vi "Single Axis Tuner.vi"() -> ()   [LabVIEW 2010]
doc: "Motor testing and tuning application for NI-73xx motion controllers. Change control loop gains, software limits, home voltage position, and other axis specific parameters on the fly for up to eight axes.\n\nDependencies:\n\nfindHome.vi\nRead Joint Angle.vi\nRead Pot.vi"
uses:
  Shared/typedefs/Trajectory Parameters.ctl
  <vilib>/Motion/FlexMotion/CustomControls/CustomControls.llb/Resource Out (Enum).flx
  <vilib>/Utility/error.llb/DialogType.ctl
  <vilib>/Motion/FlexMotion/CustomControls/CustomControls.llb/ControlGainParameter.flx
  <vilib>/Motion/FlexMotion/FunctionsVIs/StartStopMotion.llb/Stop Motion (8 axes).flx
panel:
  in  "Home Accel (RPS/s)":dbl=4.0 format="%.2f"
  in  "Home Velocity (RPM)":i32=65
  in  "Target Positions (Encoder Counts)":i32[](array[numeric])
  in  "Plot Offset":i32 step=500
  in  "Stop Type":u16(ring) items=["Decelerate", "Halt", "Kill"]
  in  "Board ID":T1=1 min=1 max=32 step=1
  in  "Reset Position":bool
  in  "Repeat Move":bool
  out "Encoder Position":i32
  out "Status Indicators":T2
  out "Desired and Actual Position v Time":T3(graph)
  out "Velocity v Time":cluster{dbl, "Position":i32}[](graph)
  out "Last Velocity":i32
  out "Last Following Error":i16=32767
  out "Following Error v Time":cluster{dbl, "Following Error":i32}[](graph)
  out "RMS Following Error":dbl
  out "Pot Value":dbl format="%#_4g"
  out "Pot Slider":dbl(slide) scale=0.0..5.0
  in  "Home Position":dbl=2.626 caption="Volts"
  in  "Axis":T4=1 items=["Axis Control"=0, "Axis 1"=1, "Axis 2"=2, "Axis 3"=3, "Axis 4"=4, "Axis 5"=5, "Axis 6"=6, "Axis 7"=7, "Axis 8"=8, "Vector Space Control"=16, "Vector Space 1"=17, "Vector Space 2"=18, "Vector Space 3"=19, "Vector Space 4"=20, "Encoder Control"=32, "Encoder 1"=33, "Encoder 2"=34, "Encoder 3"=35, "Encoder 4"=36, "Encoder 5"=37, "Encoder 6"=38, "Encoder 7"=39, "Encoder 8"=40, "DAC Channel 1"=49, "DAC Channel 2"=50, "DAC Channel 3"=51, "DAC Channel 4"=52, "DAC Channel 5"=53, "DAC Channel 6"=54, "DAC Channel 7"=55, "DAC Channel 8"=56, "Stepper Output 1"=65, "Stepper Output 2"=66, "Stepper Output 3"=67, "Stepper Output 4"=68, "Stepper Output 5"=69, "Stepper Output 6"=70, "Stepper Output 7"=71, "Stepper Output 8"=72, "ADC Channel 1"=81, "ADC Channel 2"=82, "ADC Channel 3"=83, "ADC Channel 4"=84, "ADC Channel 5"=85, "ADC Channel 6"=86, "ADC Channel 7"=87, "ADC Channel 8"=88]
  in  "Reverse SW Limit":i32=-27000 caption="Counts"
  in  "Forward SW Limit":i32=27000 caption="Counts"
  in  "Go Home":bool
  in  "Kill":bool
  in  "end program":bool
  in  "Control Gains":cluster{"Kp":u16, "Ki":u16, "Kd":u16}={"Kp"=25, "Ki"=3, "Kd"=7000}
  in  "Start":bool
  in  "Trajectory Parameters":T5={"Operation Mode (Absolute)"=0, "Blend"=FALSE, "Velocity"=6.0, "Acceleration"=4.0, "Deceleration"=4.0, "Blend Factor"=0, "Permitted Following Error"=1000.0, "S Curve Time"=0} {"Operation Mode (Absolute)" items=["Absolute Position", "Relative Position"]; "Velocity" min=0.0 max=500.0 step=1.0}
  # "NOTE: Set Board ID before beginning program execution"
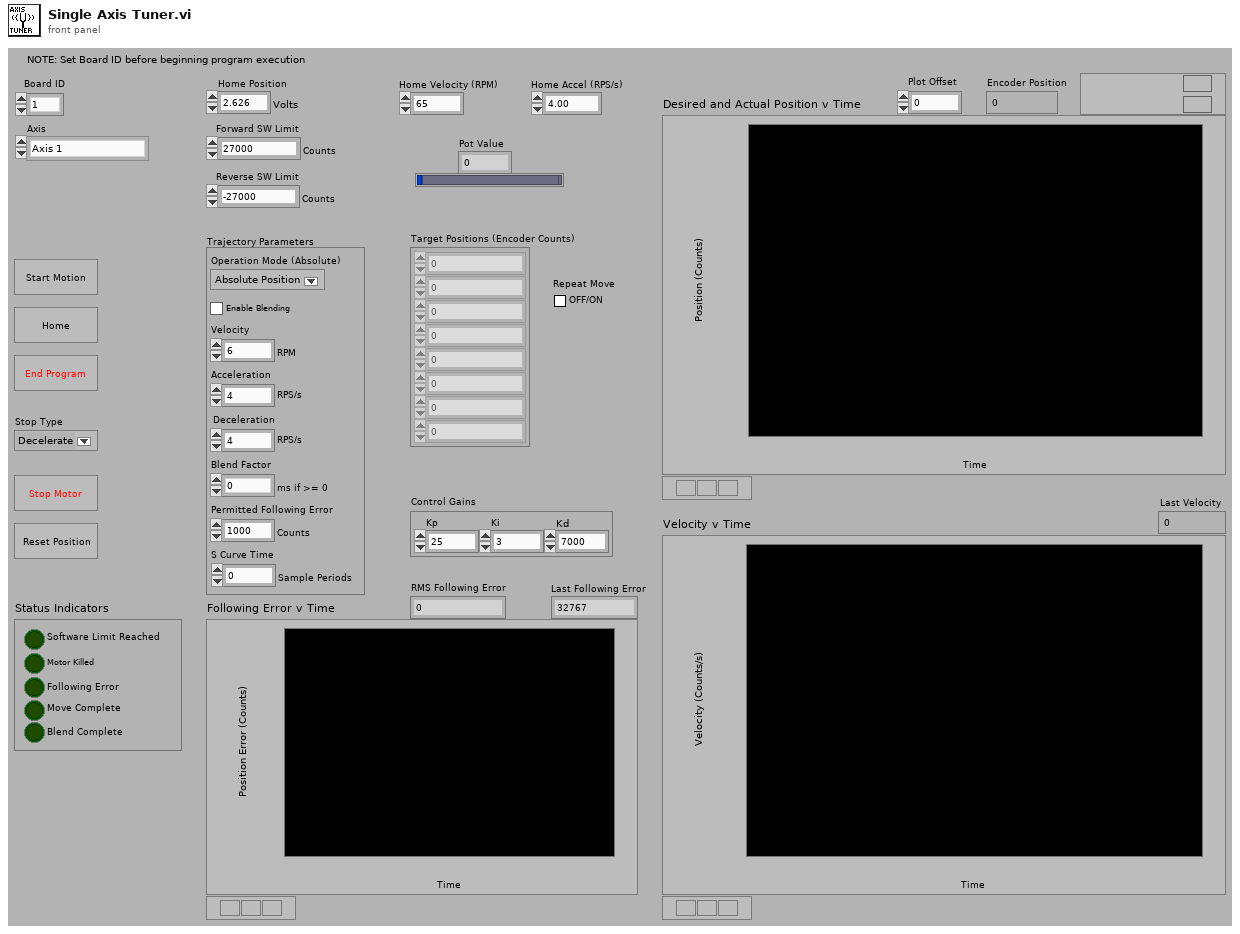
[diagram p1: front panel]
types:
  T1 = typedef "Board Id" = u8
  T2 = cluster{"Software Limit Reached":bool, "Motor Killed":bool, "Following Error":bool, "Move Complete":bool, "Blend Complete":bool}
  T3 = cluster{cluster{dbl, "Encoder Position":i32}[]}[]
  T4 = typedef "Resource Out (Enum).flx" = u16
  T5 = typedef "Trajectory Parameters.ctl" = cluster{"Operation Mode (Absolute)":u16, "Blend":bool, "Velocity":dbl, "Acceleration":dbl, "Deceleration":dbl, "Blend Factor":i16, "Permitted Following Error":dbl, "S Curve Time":u16}
  T6 = typedef "DialogType.ctl" = u16
  T7 = typedef "Bd Id Out" = u8
  T8 = cluster{"Ready to Receive":bool, "Return Data Pending":bool, "Reserved":bool, "CIP":bool, "Packet Error":bool, "Power Up Reset":bool, "Error Message":bool, "Hardware Fail":bool}
  T9 = typedef "ControlGainParameter.flx" = enum16{"Kp", "Ki", "IL", "Kd", "Td", "Kv", "Aff", "Vff"}
  T10 = enum8{"Enabled", "Disabled", "Disabled and Grayed Out"}
  T11 = typedef "Axis To Control.flx" = u16
  T12 = cluster{"Run/Stop":bool, "Profile Complete":bool, "Motor Off ":bool, "Following Error":bool, "Limit Switch":bool, "Home Switch":bool, "SW Limit Switch":bool, "Watchdog":bool, "Velocity Threshold":bool, "Position Brkpt":bool, "Home Found":bool, "Index Found":bool, "High Speed Capture":bool, "Reverse Direction":bool, "Blend Complete":bool, "Move Complete":bool}
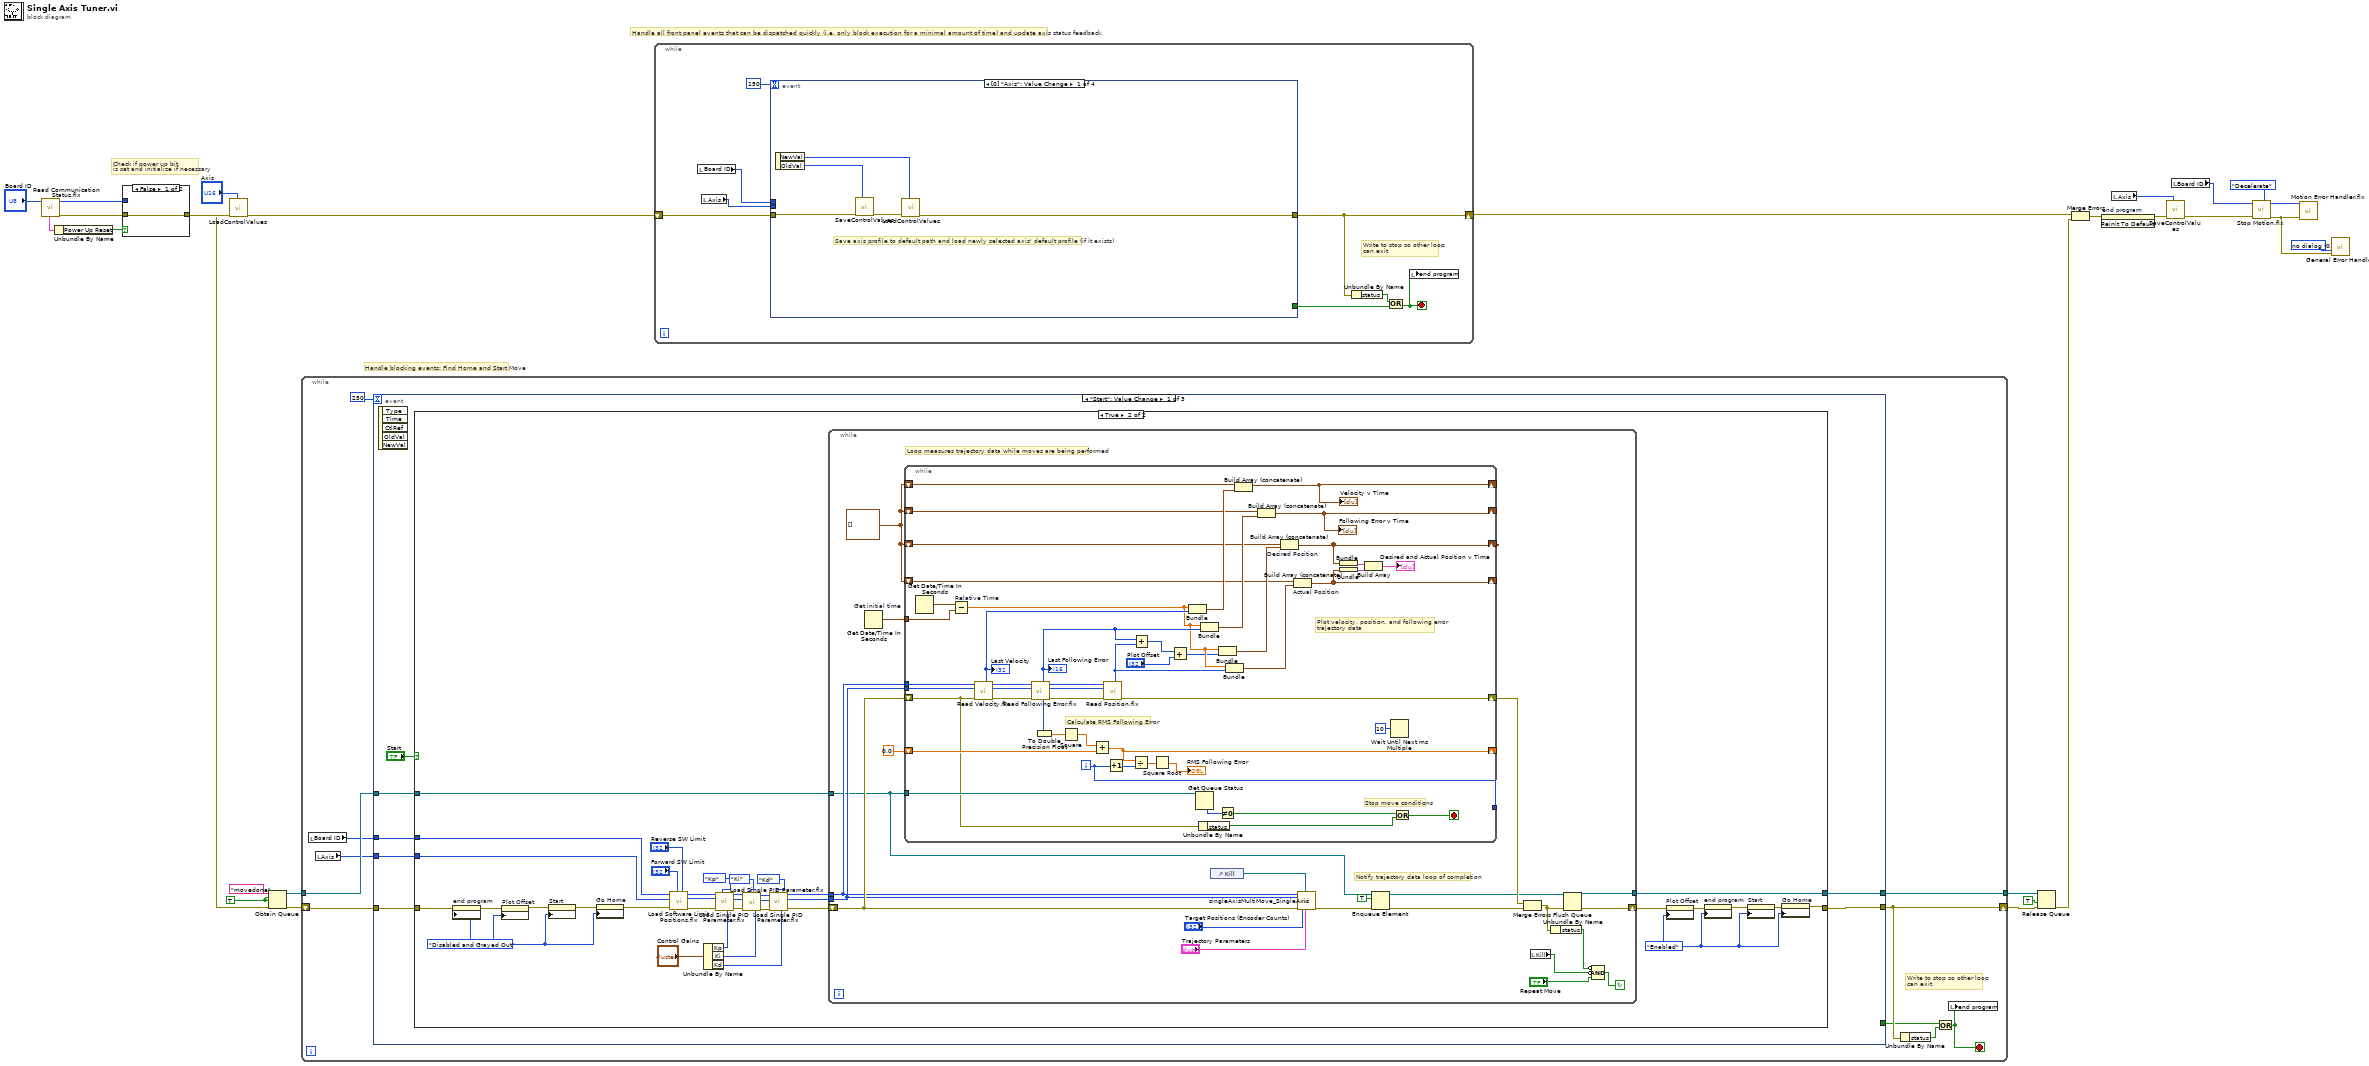
[diagram p0: block diagram]
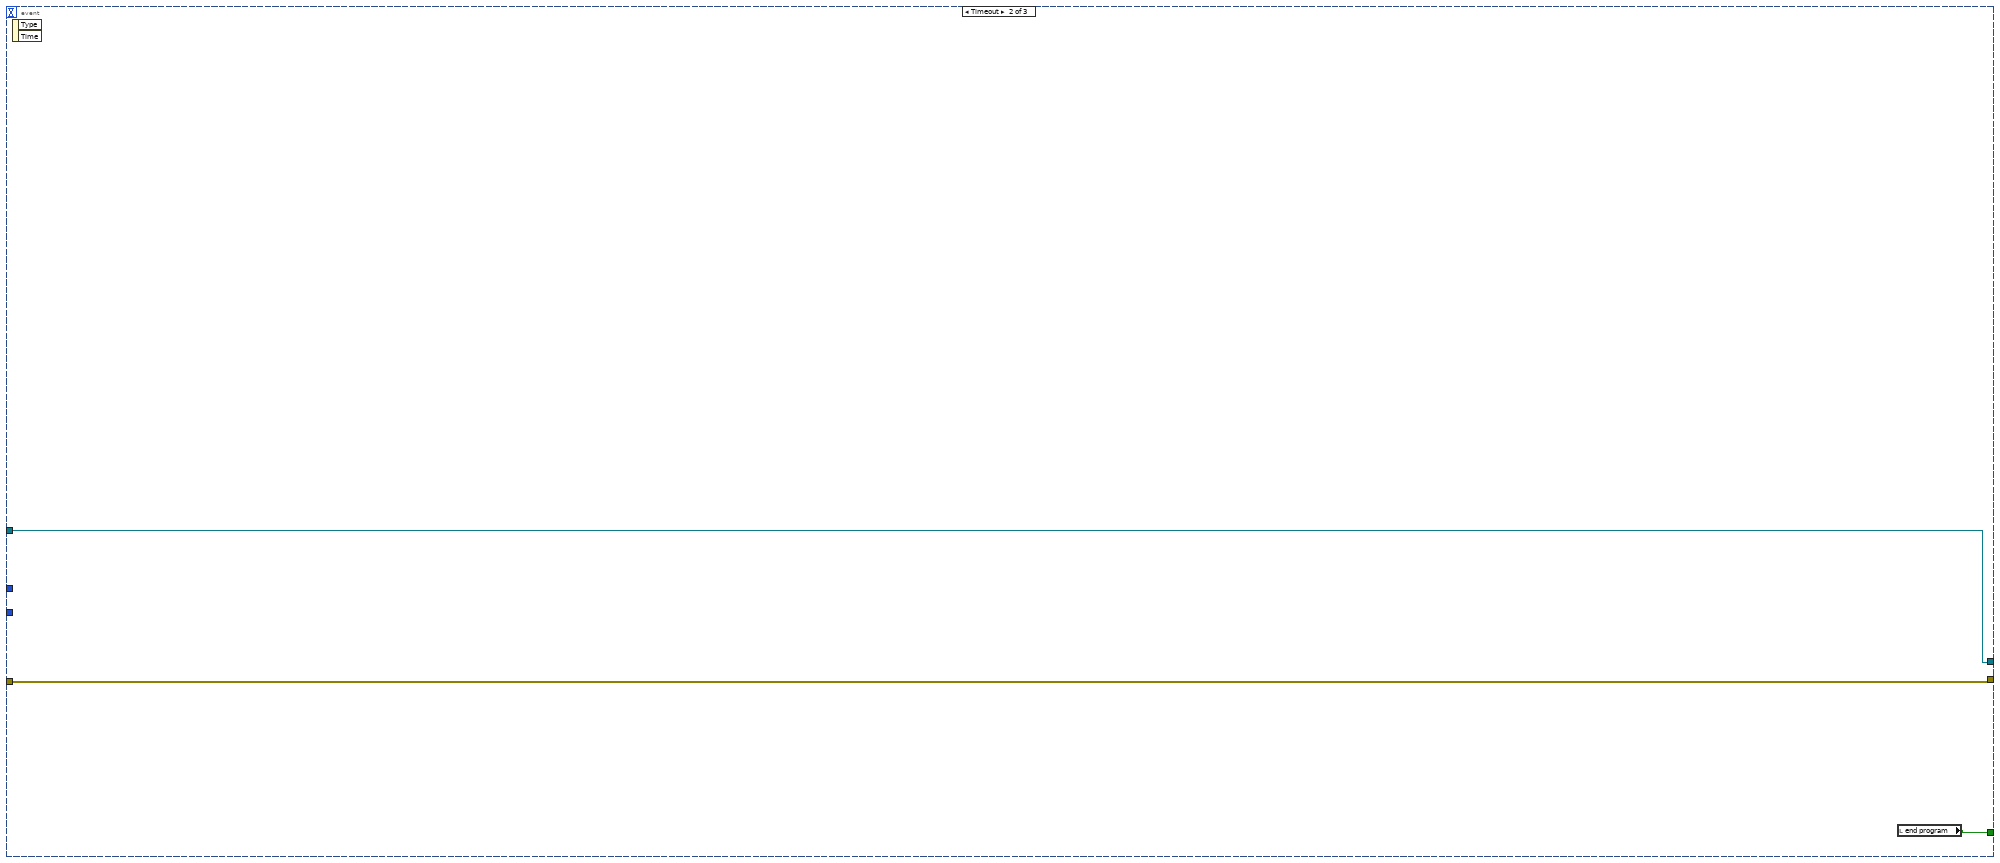
[diagram p3: hidden frame]
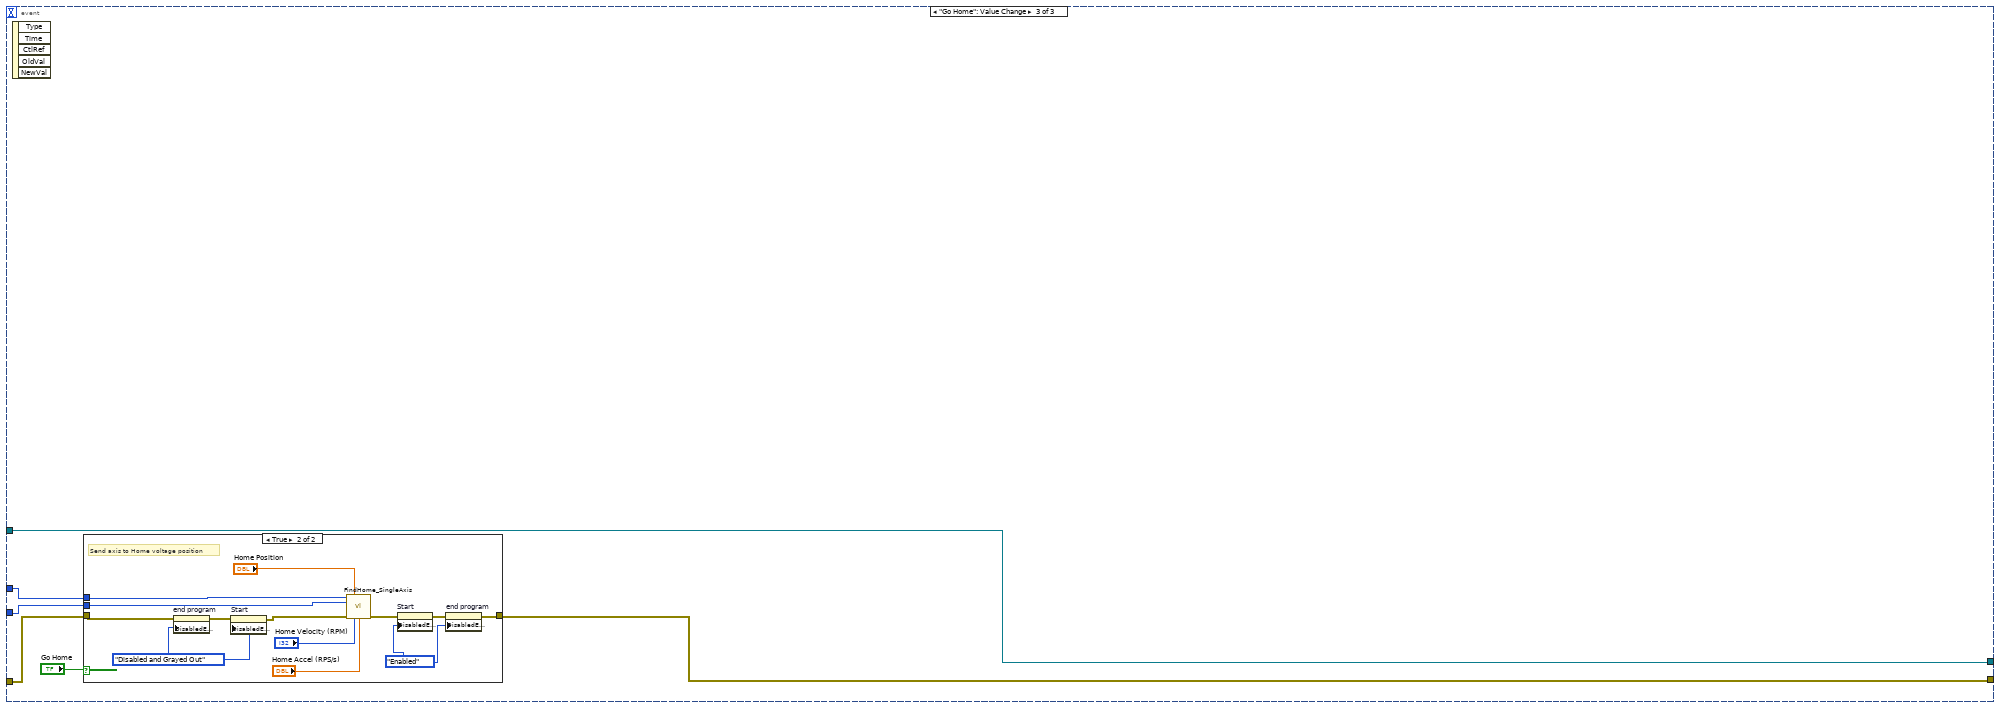
[diagram p4: hidden frame]
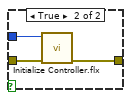
[diagram p6: hidden frame]
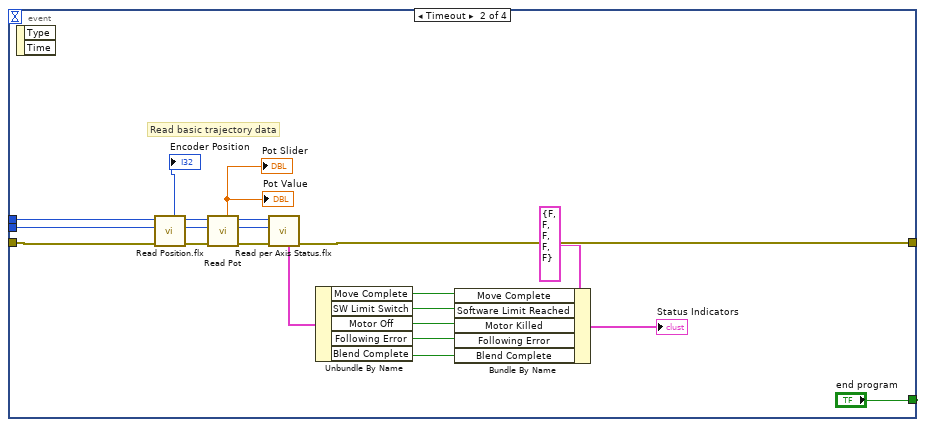
[diagram p7: hidden frame]
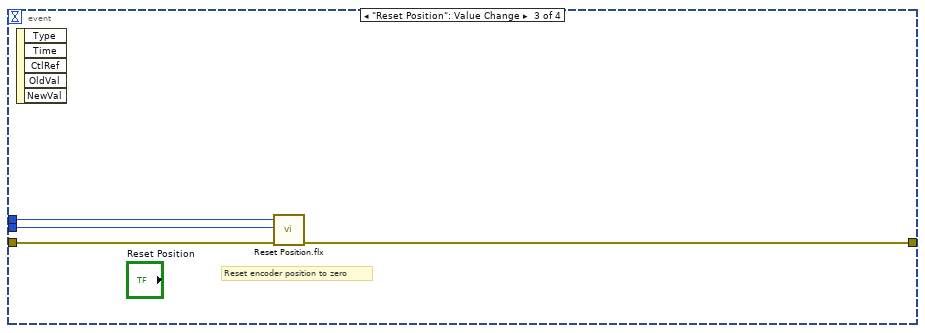
[diagram p8: hidden frame]
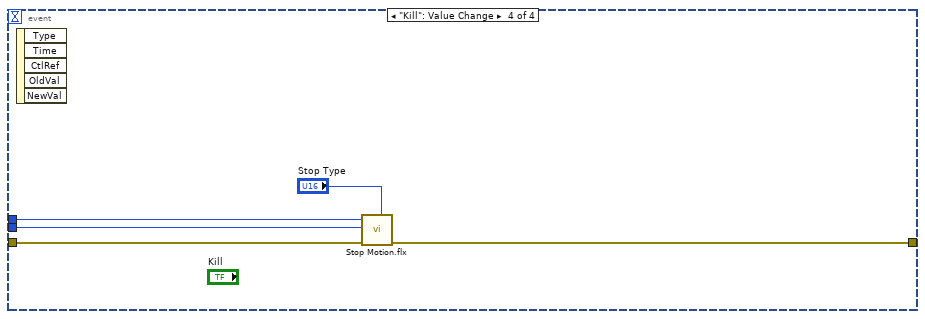
[diagram p9: hidden frame]
diagram:
  w15 = TRUE ("create if not found? (T)")
  w17 = T6 0 items=["no dialog", "OK message", "continue or stop message", "OK message + warnings", "continue/stop + warnings"] ("type of dialog (OK msg:1)")
  # "Handle blocking events: Find Home and Start Move"
  # "Handle all front panel events that can be dispatched quickly (i.e. only block execution for a minimal amount of time) and update axis status feedback."
  # "Check if power up bit\nis set and initialize if necessary"
  n1 = call <vilib>:"Read Communication Status.flx"("Board ID"="Board ID") -> ("error out"=w21:errorcluster, "Bd ID Out"=w20:T7, "Communication Status Register"=w24:T8)  [unwired: 5 in]
  n2 = Unbundle By Name(w24) -> ("Power Up Reset"=w23:bool)
  n3 = case shown="False" w23 {
    tunnel: w21 -> [w27 w29]
    tunnel: [w27 w28] -> w19
    tunnel: w20 -> [_ w30]
    frame False {
    }
    frame True {
      n4 = call <vilib>:"Initialize Controller.flx"("error in (no error)"=w29, "Board ID"=w30) -> ("error out"=w28:errorcluster)  [unwired: 6 in, 1 out]
    }
  }
  n5 = call "LoadControlValues.vi"("Axis"="Axis", "error in (no error)"=w19) -> ("error out"=w10:errorcluster)  [unwired: 9 in]
  n6 = Obtain Queue(name (unnamed)="movedone", element data type=w15, create if not found? (T)=w15, error in (no error)=w10) -> (queue out=w11:refnum<queue>, error out=w14:errorcluster)  [unwired: 1 in, 1 out]
  n7 = while {
    shift-right: [w39] -> w2
    shift-left: w14 -> [w40]
    tunnel: w11 -> [w37]
    tunnel: [w31] -> w1
    stop <- w38 stop-if-true
    # "Write to stop so other loop\ncan exit"
    n8 = local read "Board ID"() -> (w35:T1)
    n9 = local read "Axis"() -> (w34:T4)
    n10 = event shown="[0] \"Start\": Value Change" {
      selector: _ -> [_ _ _]
      dyn-events: _ -> [_ _ _]
      timeout: 250 -> [_ _ _]
      tunnel: w40 -> [w47 w157 w162]
      tunnel: [w46 w157 w161] -> w39
      tunnel: w37 -> [w45 w158 w160]
      tunnel: [w44 w158 w160] -> w31
      tunnel: [_ w159 _] -> w32
      tunnel: w35 -> [w42 _ w164]
      tunnel: w34 -> [w41 _ w163]
      event "Start": Value Change {
        n11 = event-data() -> ()  [unwired: 1 in, 5 out]
        n12 = case shown="True" "Start" {
          tunnel: [w49 w54] -> w46
          tunnel: w47 -> [w49 w64]
          tunnel: w45 -> [w48 w65]
          tunnel: [w48 w52] -> w44
          tunnel: w42 -> [_ w51]
          tunnel: w41 -> [_ w50]
          frame False {
          }
          frame True {
            w53 = T10."Enabled" ("Disabled")
            w56 = T10."Disabled and Grayed Out" ("Disabled")
            n13 = property on="end program" class="Bool (strict)"(error in=w64, "DisabledEnum"=w56) -> (error out=w63:errorcluster)  [unwired: 1 in, 1 out]
            n14 = property on="Plot Offset" class="DigNum (strict)"(error in=w63, "DisabledEnum"=w56) -> (error out=w60:errorcluster)  [unwired: 1 in, 1 out]
            n15 = property on="Start" class="Bool"(error in=w60, "DisabledEnum"=w56) -> (error out=w58:errorcluster)  [unwired: 1 in, 1 out]
            n16 = property on="Go Home" class="Bool"(error in=w58, "DisabledEnum"=w56) -> (error out=w57:errorcluster)  [unwired: 1 in, 1 out]
            n17 = call <vilib>:"Load Software Limit Positions.flx"("Reverse SW Limit"="Reverse SW Limit", "Forward SW Limit"="Forward SW Limit", "error in (no error)"=w57, "Axis"=w50, "Board ID"=w51) -> ("error out"=w73:errorcluster, "Resource Output"=w72:T4, "Bd ID Out"=w71:T7)  [unwired: 2 in]
            n18 = Unbundle By Name("Control Gains") -> ("Kp"=w76:u16, "Ki"=w75:u16, "Kd"=w74:u16)
            n19 = call <vilib>:"Load Single PID Parameter.flx"("Value (0)"=w76, "Parameter (Kp)"=ControlGainParameter.flx."Kp", "error in (no error)"=w73, "Axis"=w72, "Board ID"=w71) -> ("error out"=w84:errorcluster, "Resource Output"=w85:T4, "Bd ID Out"=w86:T7)  [unwired: 2 in]
            n20 = call <vilib>:"Load Single PID Parameter.flx"("Value (0)"=w75, "Parameter (Kp)"=ControlGainParameter.flx."Ki", "error in (no error)"=w84, "Axis"=w85, "Board ID"=w86) -> ("error out"=w81:errorcluster, "Resource Output"=w82:T4, "Bd ID Out"=w83:T7)  [unwired: 2 in]
            n21 = call <vilib>:"Load Single PID Parameter.flx"("Value (0)"=w74, "Parameter (Kp)"=ControlGainParameter.flx."Kd", "error in (no error)"=w81, "Axis"=w82, "Board ID"=w83) -> ("error out"=w68:errorcluster, "Resource Output"=w66:T4, "Bd ID Out"=w67:T7)  [unwired: 2 in]
            n22 = while {
              shift-right: [w95] -> w61
              shift-left: w68 -> [w105]
              tunnel: w67 -> [w104]
              tunnel: w66 -> [w103]
              tunnel: w65 -> [w100]
              tunnel: [w92] -> w52
              stop <- w98 continue-if-true
              w106 = cluster{dbl, i32}[] [] ("XY Graph")
              # "Loop measures trajectory data while moves are being performed"
              # "Notify trajectory data loop of completion"
              n23 = Get Date/Time In Seconds "Get initial time"() -> (seconds since 1Jan1904=w107:timestamp)
              n24 = while {
                tunnel: w107 -> [w156]
                shift-right: [w126] -> _
                shift-left: w106 -> [w128]
                shift-right: [w116] -> w96
                shift-left: w105 -> [w109]
                shift-right: [w152] -> _
                shift-left: w106 -> [w151]
                shift-right: [w148] -> _
                shift-left: w106 -> [w150]
                shift-right: [w144] -> _
                shift-left: 0.0 -> [w140]
                tunnel: [w119] -> _
                shift-right: [w127] -> _
                shift-left: w106 -> [w129]
                tunnel: w104 -> [w111]
                tunnel: w103 -> [w110]
                tunnel: w100 -> [w118]
                i -> [w119]
                stop <- w113 stop-if-true
                # "Stop move conditions"
                # "Plot velocity, position, and following error \ntrajectory data"
                # "Calculate RMS Following Error"
                n25 = Get Date/Time In Seconds ("Get Current Time")() -> (seconds since 1Jan1904=w155:timestamp)
                n26 = Subtract "Relative Time"(x=w155, y=w156) -> (x-y=w123:dbl)
                n27 = call <vilib>:"Read Velocity.flx"("error in (no error)"=w109, "Axis or Vector Space"=w110, "Board ID"=w111) -> ("error out"=w137:errorcluster, "Resource Output"=w135:T4, "Bd ID Out"=w136:T7, "Filtered Velocity"=w154:i32)  [unwired: 3 in]
                "Last Velocity" <- w154
                n28 = call <vilib>:"Read Following Error.flx"("error in (no error)"=w137, "Axis or Vector Space"=w135, "Board Id"=w136) -> ("error out"=w132:errorcluster, "Resource Output"=w133:T4, "Bd Id Out"=w134:T7, "Following Error"=w139:i16)  [unwired: 3 in]
                "Last Following Error" <- w139
                n29 = To Double Precision Float(number=w139) -> (double precision float=w143:dbl)
                n30 = Square(x=w143) -> (x^2=w141:dbl)
                n31 = Add(x=w141, y=w140) -> (x+y=w144:dbl)
                n32 = call <vilib>:"Read Position.flx"("error in (no error)"=w132, "Axis"=w133, "Board ID"=w134) -> ("error out"=w116:errorcluster, "Position"=w131:i32)  [unwired: 3 in, 2 out]
                n33 = Increment(x=w119) -> (x+1=w147:i32)
                n34 = Divide(x=w144, y=w147) -> (x/y=w145:dbl)
                n35 = Add(x=w139, y=w131) -> (x+y=w122:i32)
                n36 = Square Root(x=w145) -> (sqrt(x)=→"RMS Following Error":dbl)
                n37 = Add(x=w122, y="Plot Offset") -> (x+y=w121:i32)
                n38 = Bundle(w123, "Filtered Velocity"=w154) -> (w153:cluster{dbl, "Filtered Velocity":i32})  [unwired: 1 in]
                n39 = Get Queue Status(queue=w118) -> (# elements in queue=w117:i32)  [unwired: 2 in, 7 out]
                n40 = Unbundle By Name(w109) -> ("status"=w112:bool)
                n41 = Bundle(w123, "Following Error"=w139) -> (w149:cluster{dbl, "Following Error":i16})  [unwired: 1 in]
                n42 = Bundle(w123, w121) -> (w130:cluster{dbl, i32})  [unwired: 1 in]
                n43 = Not Equal To 0?(x=w117) -> (x != 0?=w114:bool)
                n44 = Bundle(w123, "Position"=w131) -> (w142:cluster{dbl, "Position":i32})  [unwired: 1 in]
                n45 = Build Array (concatenate)(w151, w153) -> (w152:cluster{dbl, "Filtered Velocity":i32}[])
                "Velocity v Time" <- w152
                n46 = Build Array (concatenate)(w150, w149) -> (w148:cluster{dbl, "Following Error":i32}[])
                "Following Error v Time" <- w148
                n47 = Build Array (concatenate) "Desired Position"(w129, w130) -> (w127:cluster{dbl, i32}[])
                n48 = Build Array (concatenate) "Actual Position"(w128, w142) -> (w126:cluster{dbl, "Position":i32}[])
                n49 = Bundle(w127) -> (w124:cluster{cluster{dbl, i32}[]})  [unwired: 1 in]
                n50 = Bundle(w126) -> (w125:cluster{cluster{dbl, "Position":i32}[]})  [unwired: 1 in]
                n51 = Build Array(w124, w125) -> (→"Desired and Actual Position v Time":cluster{cluster{dbl, "Position":i32}[]}[])
                n52 = Wait Until Next ms Multiple(millisecond multiple=u32 10) -> ()  [unwired: 1 out]
                n53 = Or(x=w114, y=w112) -> (x .or. y?=w113:bool)
              }
              n54 = control-ref of="Kill"() -> (w93:refnum<vi>)
              n55 = call "singleAxisMultiMove_SingleAxis.vi"("Bd ID"=w104, "Axis"=w103, "error in (no error)"=w105, "Target Positions"="Target Positions (Encoder Counts)", "Stop Refnum"=w93, "Trajectory Parameters"="Trajectory Parameters") -> ("error out"=w99:errorcluster)  [unwired: 11 in, 2 out]
              n56 = Enqueue Element(queue=w100, element=TRUE, error in (no error)=w99) -> (queue out=w94:refnum<queue>, error out=w97:errorcluster)  [unwired: 1 in, 1 out]
              n57 = Merge Errors(w96, w97) -> (w91:errorcluster)
              n58 = local read "Kill"() -> (w88:bool)
              n59 = Unbundle By Name(w91) -> ("status"=w90:bool)
              n60 = Flush Queue(queue=w94, error in (no error)=w91) -> (queue out=w92:refnum<queue>, error out=w95:errorcluster)  [unwired: 1 out]
              n61 = Compound Arithmetic op=AND(invert w90, invert w88, "Repeat Move") -> (w98:bool)
            }
            n62 = property on="Plot Offset" class="DigNum (strict)"(error in=w61, "DisabledEnum"=w53) -> (error out=w62:errorcluster)  [unwired: 1 in, 1 out]
            n63 = property on="end program" class="Bool (strict)"(error in=w62, "DisabledEnum"=w53) -> (error out=w59:errorcluster)  [unwired: 1 in, 1 out]
            n64 = property on="Start" class="Bool"(error in=w59, "DisabledEnum"=w53) -> (error out=w55:errorcluster)  [unwired: 1 in, 1 out]
            n65 = property on="Go Home" class="Bool"(error in=w55, "DisabledEnum"=w53) -> (error out=w54:errorcluster)  [unwired: 1 in, 1 out]
          }
        }
      }
      event Timeout {
        n66 = event-data() -> ()  [unwired: 1 in, 2 out]
        n67 = local read "end program"() -> (w159:bool)
      }
      event "Go Home": Value Change {
        n68 = event-data() -> ()  [unwired: 1 in, 5 out]
        n69 = case shown="True" "Go Home" {
          tunnel: w162 -> [w166 w174]
          tunnel: [w166 w170] -> w161
          tunnel: w164 -> [_ w179]
          tunnel: w163 -> [_ w178]
          frame False {
          }
          frame True {
            w171 = T10."Enabled" ("Disabled")
            w173 = T10."Disabled and Grayed Out" ("Disabled")
            # "Send axis to Home voltage position"
            n70 = property on="end program" class="Bool (strict)"(error in=w174, "DisabledEnum"=w173) -> (error out=w175:errorcluster)  [unwired: 1 in, 1 out]
            n71 = property on="Start" class="Bool"(error in=w175, "DisabledEnum"=w173) -> (error out=w176:errorcluster)  [unwired: 1 in, 1 out]
            n72 = call "FindHome_SingleAxis.vi"("Bd ID In"=w179, "Home Voltage"="Home Position", "Axis"=w178, "error in"=w176, "Velocity (RPM)"="Home Velocity (RPM)", "Acceleration (RPS/s)"="Home Accel (RPS/s)") -> ("error out"=w169:errorcluster)  [unwired: 7 in, 2 out]
            n73 = property on="Start" class="Bool"(error in=w169, "DisabledEnum"=w171) -> (error out=w172:errorcluster)  [unwired: 1 in, 1 out]
            n74 = property on="end program" class="Bool (strict)"(error in=w172, "DisabledEnum"=w171) -> (error out=w170:errorcluster)  [unwired: 1 in, 1 out]
          }
        }
      }
    }
    n75 = Unbundle By Name(w39) -> ("status"=w33:bool)
    n76 = Or(x=w32, y=w33) -> (x .or. y?=w38:bool)
    n77 = local write "end program"(w38) -> ()
  }
  n78 = while {
    shift-right: [w184] -> w5
    shift-left: w10 -> [w186]
    stop <- w182 stop-if-true
    # "Write to stop so other loop\ncan exit"
    n79 = local read "Board ID"() -> (w185:T1)
    n80 = local read "Axis"() -> (w181:T4)
    n81 = event shown="[0] \"Axis\": Value Change" {
      selector: _ -> [_ _ _ _]
      dyn-events: _ -> [_ _ _ _]
      timeout: u32 150 ("millisecond multiple") -> [_ _ _ _]
      tunnel: [w188 w195 w214 w219] -> w184
      tunnel: w186 -> [w190 w200 w215 w220]
      tunnel: w181 -> [_ w201 w216 w221]
      tunnel: w185 -> [_ w202 w217 w222]
      tunnel: [_ "end program" _ _] -> w180
      event Value Change {
        # "Save axis profile to default path and load newly selected axis' default profile (if it exists)"
        n82 = event-data() -> ("NewVal"=w191:T4, "OldVal"=w192:T4)  [unwired: 1 in]
        n83 = call "SaveControlValues.vi"("Axis"=w192, "error in"=w190) -> ("error out"=w189:errorcluster)  [unwired: 7 in]
        n84 = call "LoadControlValues.vi"("Axis"=w191, "error in (no error)"=w189) -> ("error out"=w188:errorcluster)  [unwired: 9 in]
      }
      event Timeout {
        # "Read basic trajectory data"
        n85 = event-data() -> ()  [unwired: 1 in, 2 out]
        n86 = call <vilib>:"Read Position.flx"("error in (no error)"=w200, "Axis"=w201, "Board ID"=w202) -> ("error out"=w203:errorcluster, "Resource Output"=w205:T4, "Bd ID Out"=w204:T7, "Position"=→"Encoder Position":i32)  [unwired: 3 in]
        n87 = call "Read Pot.vi"("error in (no error)"=w203, "Axis In"=w205, "Board ID"=w204) -> ("error out"=w212:errorcluster, "Axis Out"=w211:T11, "Bd ID Out"=w210:T7, "Pot Voltage"=→"Pot Value" →"Pot Slider":dbl)  [unwired: 5 in]
        n88 = call <vilib>:"Read per Axis Status.flx"("error in (no error)"=w212, "Axis"=w211, "Board ID"=w210) -> ("error out"=w195:errorcluster, "Per Axis H/W Status"=w206:T12)  [unwired: 3 in, 2 out]
        n89 = Unbundle By Name(w206) -> ("Move Complete"=w213:bool, "SW Limit Switch"=w208:bool, "Motor Off"=w207:bool, "Following Error"=w209:bool, "Blend Complete"=w198:bool)
        n90 = Bundle By Name(cluster=T2 {"Software Limit Reached"=FALSE, "Motor Killed"=FALSE, "Following Error"=FALSE, "Move Complete"=FALSE, "Blend Complete"=FALSE} ("Status Indicators"), "Move Complete"=w213, "Software Limit Reached"=w208, "Motor Killed"=w207, "Following Error"=w209, "Blend Complete"=w198) -> (→"Status Indicators":T2)
      }
      event "Reset Position": Value Change {
        # "Reset encoder position to zero"
        n91 = event-data() -> ()  [unwired: 1 in, 5 out]
        n92 = call <vilib>:"Reset Position.flx"("error in (no error)"=w215, "Axis"=w216, "Board ID"=w217) -> ("error out"=w214:errorcluster)  [unwired: 4 in, 2 out]
      }
      event "Kill": Value Change {
        n93 = event-data() -> ()  [unwired: 1 in, 5 out]
        n94 = call-poly <vilib>:"Stop Motion.flx"("Stop Type (Decel)"="Stop Type", "error in (no error)"=w220, "Axis or Vector Space"=w221, "Board ID"=w222) -> ("error out"=w219:errorcluster)  [unwired: 3 in, 2 out]
      }
    }
    n95 = Unbundle By Name(w184) -> ("status"=w187:bool)
    n96 = Compound Arithmetic op=OR(w187, w180) -> (w182:bool)
    n97 = local write "end program"(w182) -> ()
  }
  n98 = Release Queue(queue=w1, force destroy? (F)=TRUE, error in (no error)=w2) -> (error out=w13:errorcluster)  [unwired: 2 out]
  n99 = Merge Errors(w5, w13) -> (w8:errorcluster)
  n100 = invoke on="end program" class="Bool (strict)" method="Reinit To Default"(error in=w8) -> (error out=w7:errorcluster)  [unwired: 2 in, 2 out]
  n101 = local read "Axis"() -> (w3:T4)
  n102 = call "SaveControlValues.vi"("Axis"=w3, "error in"=w7) -> ("error out"=w6:errorcluster)  [unwired: 7 in]
  n103 = local read "Board ID"() -> (w18:T1)
  n104 = call-poly <vilib>:"Stop Motion.flx"("Stop Type (Decel)"=enum16{"Decelerate", "Halt", "Kill"}."Decelerate", "error in (no error)"=w6, "Board ID"=w18) -> ("error out"=w9:errorcluster, "Bd ID Out"=w26:T7)  [unwired: 4 in, 1 out]
  n105 = call <vilib>:"Motion Error Handler.flx"("Board ID"=w26, "error in (no error)"=w9) -> ()  [unwired: 9 in, 5 out]
  n106 = call <vilib>:"General Error Handler.vi"("type of dialog (OK msg:1)"=w17, "error in (no error)"=w9) -> ()  [unwired: 9 in, 5 out]
